vi "Get Limits.vi"(11 "Limits File Path":path=path "D:/PR002165_FCT_NGPMH/UTP/misc/Limits/Production_Limits.csv") -> (2 "DUT2":T1, 3 "DUT1":T1)   [LabVIEW 2023]
uses:
  DUT limits.ctl
  <vilib>/Utility/file.llb/Read Delimited Spreadsheet (DBL).vi
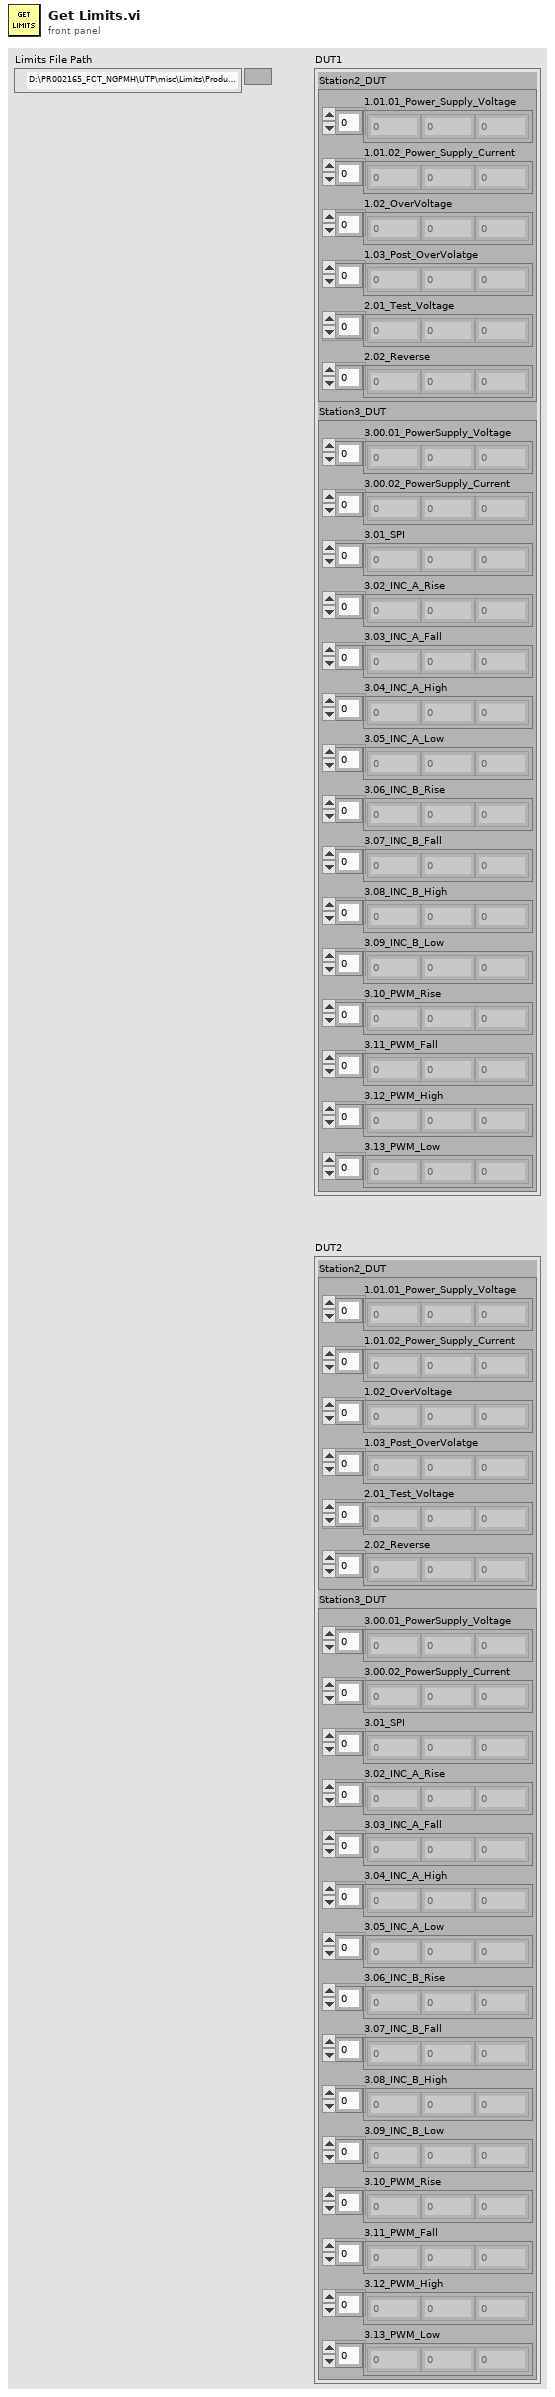
[diagram p1: front panel]
types:
  T1 = typedef "DUT limits.ctl" = cluster{"Station2_DUT":cluster{"1.01.01_Power_Supply_Voltage":dbl[], "1.01.02_Power_Supply_Current":dbl[], "1.02_OverVoltage":dbl[], "1.03_Post_OverVolatge":dbl[], "2.01_Test_Voltage":dbl[], "2.02_Reverse":dbl[]}, "Station3_DUT":cluster{"3.00.01_PowerSupply_Voltage":dbl[], "3.00.02_PowerSupply_Current":dbl[], "3.01_SPI":dbl[], "3.02_INC_A_Rise":dbl[], "3.03_INC_A_Fall":dbl[], "3.04_INC_A_High":dbl[], "3.05_INC_A_Low":dbl[], "3.06_INC_B_Rise":dbl[], "3.07_INC_B_Fall":dbl[], "3.08_INC_B_High":dbl[], "3.09_INC_B_Low":dbl[], "3.10_PWM_Rise":dbl[], "3.11_PWM_Fall":dbl[], "3.12_PWM_High":dbl[], "3.13_PWM_Low":dbl[]}}
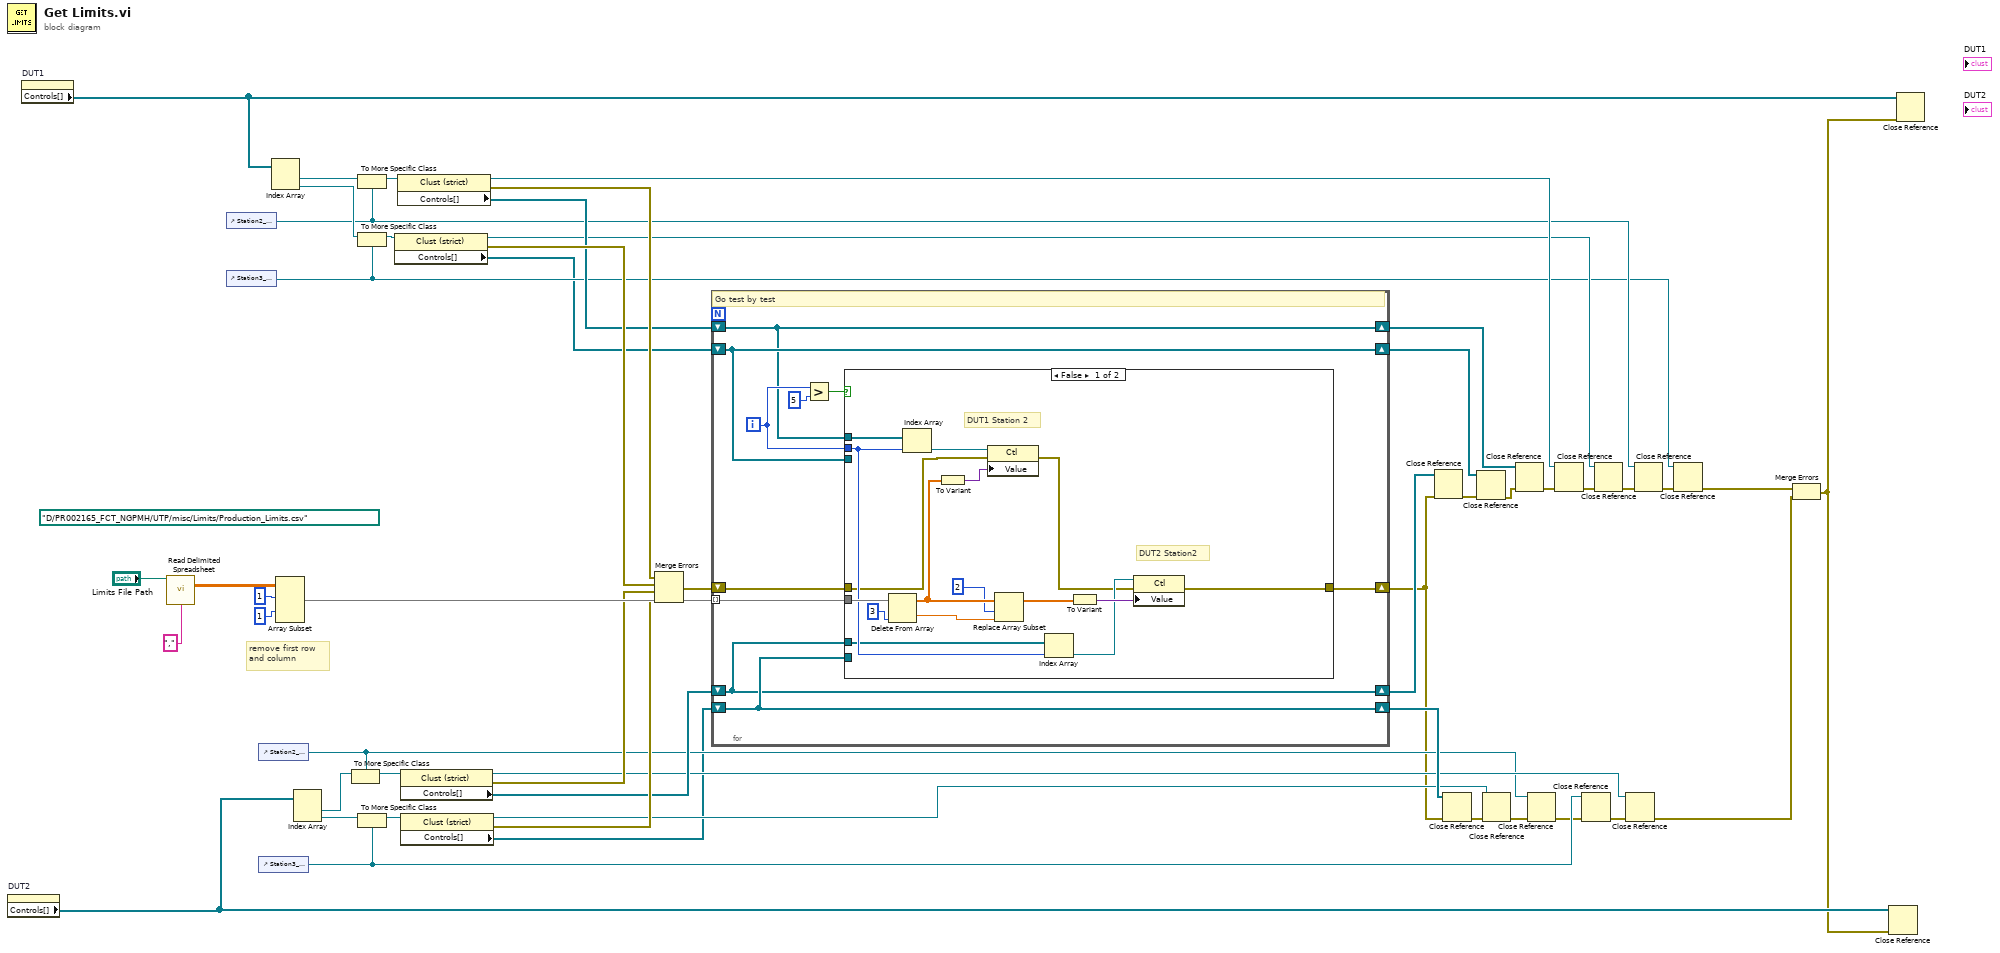
[diagram p0: block diagram]
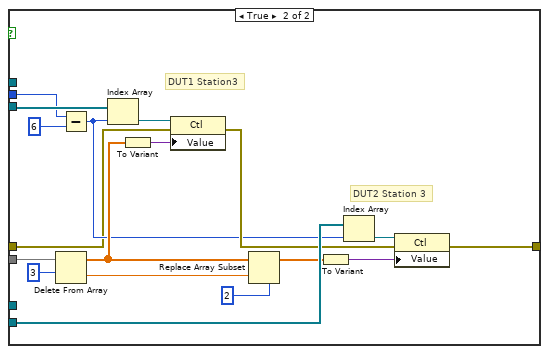
[diagram p2: hidden frame]
diagram:
  (unwired) path "D:/PR002165_FCT_NGPMH/UTP/misc/Limits/Production_Limits.csv" ("file path (dialog if empty)")
  # "remove first row\nand column"
  n1 = property on="DUT2" class="Clust (strict)"() -> ("Controls[]"=w27:refnum<vi>[])  [unwired: 2 in, 2 out]
  n2 = property on="DUT1" class="Clust (strict)"() -> ("Controls[]"=w11:refnum<vi>[])  [unwired: 2 in, 2 out]
  n3 = call-poly <vilib>:"Read Delimited Spreadsheet.vi"("file path (dialog if empty)"="Limits File Path", "delimiter (\\t)"="," ("delimiter (\\t)")) -> ("all rows"=w50:dbl[][])  [unwired: 8 in, 5 out]
  n4 = control-ref of="Station2_DUT"() -> (w19:refnum<vi>)
  n5 = control-ref of="Station3_DUT"() -> (w17:refnum<vi>)
  n6 = control-ref of="Station2_DUT"() -> (w15:refnum<vi>)
  n7 = control-ref of="Station3_DUT"() -> (w14:refnum<vi>)
  n8 = Index Array(array=w11) -> (element #1=w46:refnum<vi>, element #2=w44:refnum<vi>)  [unwired: 2 in]
  n9 = Array Subset(array=w50, index (row)=1 ("index"), index (col)=1 ("index")) -> (w48:dbl[][])  [unwired: 2 in]
  n10 = Index Array(array=w27) -> (element #1=w41:refnum<vi>, element #2=w40:refnum<vi>)  [unwired: 2 in]
  n11 = To More Specific Class(target class=w15, reference=w41) -> (specific class reference=w39:refnum<vi>)  [unwired: 1 in, 1 out]
  n12 = To More Specific Class(target class=w19, reference=w46) -> (specific class reference=w47:refnum<vi>)  [unwired: 1 in, 1 out]
  n13 = To More Specific Class(target class=w17, reference=w44) -> (specific class reference=w45:refnum<vi>)  [unwired: 1 in, 1 out]
  n14 = To More Specific Class(target class=w14, reference=w40) -> (specific class reference=w38:refnum<vi>)  [unwired: 1 in, 1 out]
  n15 = property class="Clust (strict)"(reference=w45) -> (reference out=w21:refnum<vi>, error out=w36:errorcluster, "Controls[]"=w5:refnum<vi>[])  [unwired: 1 in]
  n16 = property class="Clust (strict)"(reference=w47) -> (reference out=w23:refnum<vi>, error out=w37:errorcluster, "Controls[]"=w24:refnum<vi>[])  [unwired: 1 in]
  n17 = property class="Clust (strict)"(reference=w39) -> (reference out=w28:refnum<vi>, error out=w35:errorcluster, "Controls[]"=w33:refnum<vi>[])  [unwired: 1 in]
  n18 = property class="Clust (strict)"(reference=w38) -> (reference out=w29:refnum<vi>, error out=w34:errorcluster, "Controls[]"=w4:refnum<vi>[])  [unwired: 1 in]
  n19 = Merge Errors(w37, w36, w35, w34) -> (w9:errorcluster)
  n20 = for {
    tunnel: w48 -> [w61] mode=indexing
    shift-right: [w57] -> w43
    shift-left: w5 -> [w57]
    shift-right: [w56] -> w42
    shift-left: w24 -> [w56]
    shift-right: [w54] -> w32
    shift-left: w33 -> [w54]
    shift-right: [w55] -> w31
    shift-left: w4 -> [w55]
    shift-right: [w53] -> w6
    shift-left: w9 -> [w52]
    i -> [w58]
    # "Go test by test"
    n21 = Greater?(x=w58, y=5) -> (0:w59:bool)
    n22 = case shown="False" w59 {
      tunnel: w57 -> [_ w95]
      tunnel: w56 -> [w65 _]
      tunnel: w58 -> [w68 w90]
      tunnel: w61 -> [w71 w88]
      tunnel: w55 -> [_ w91]
      tunnel: w54 -> [w64 _]
      tunnel: [w63 w80] -> w53
      tunnel: w52 -> [w62 w78]
      frame False {
        # "DUT1 Station 2"
        # "DUT2 Station2"
        n23 = Delete From Array(array=w71, index=3 ("length")) -> (deleted portion=w73:dbl, array with subset deleted=w75:dbl[])  [unwired: 1 in]
        n24 = Index Array(array=w65, index=w68) -> (element=w77:refnum<vi>)
        n25 = To Variant(anything=w75) -> (Variant=w70:variant)
        n26 = property class="Ctl"(reference=w77, error in=w62, "Value"=w70) -> (error out=w66:errorcluster)  [unwired: 1 out]
        n27 = Replace Array Subset(array=w75, new element=w73, index=2) -> (w72:dbl[])
        n28 = Index Array(array=w64, index=w68) -> (element=w67:refnum<vi>)
        n29 = To Variant(anything=w72) -> (Variant=w69:variant)
        n30 = property class="Ctl"(reference=w67, error in=w66, "Value"=w69) -> (error out=w63:errorcluster)  [unwired: 1 out]
      }
      frame True {
        # "DUT1 Station3"
        # "DUT2 Station 3"
        n31 = Delete From Array(array=w88, index=3 ("length")) -> (deleted portion=w84:dbl, array with subset deleted=w86:dbl[])  [unwired: 1 in]
        n32 = Subtract(x=w90, y=6) -> (x-y=w79:i32)
        n33 = Index Array(array=w95, index=w79) -> (element=w93:refnum<vi>)
        n34 = To Variant(anything=w86) -> (Variant=w92:variant)
        n35 = property class="Ctl"(reference=w93, error in=w78, "Value"=w92) -> (error out=w81:errorcluster)  [unwired: 1 out]
        n36 = Replace Array Subset(array=w86, new element=w84, index=2) -> (w83:dbl[])
        n37 = To Variant(anything=w83) -> (Variant=w82:variant)
        n38 = Index Array(array=w91, index=w79) -> (element=w89:refnum<vi>)
        n39 = property class="Ctl"(reference=w89, error in=w81, "Value"=w82) -> (error out=w80:errorcluster)  [unwired: 1 out]
      }
    }
  }
  n40 = Close Reference(reference=w32, error in (no error)=w6) -> (error out=w7:errorcluster)
  n41 = Close Reference(reference=w31, error in (no error)=w6) -> (error out=w30:errorcluster)
  n42 = Close Reference(reference=w43, error in (no error)=w7) -> (error out=w8:errorcluster)
  n43 = Close Reference(reference=w29, error in (no error)=w30) -> (error out=w2:errorcluster)
  n44 = Close Reference(reference=w42, error in (no error)=w8) -> (error out=w22:errorcluster)
  n45 = Close Reference(reference=w15, error in (no error)=w2) -> (error out=w13:errorcluster)
  n46 = Close Reference(reference=w23, error in (no error)=w22) -> (error out=w20:errorcluster)
  n47 = Close Reference(reference=w14, error in (no error)=w13) -> (error out=w1:errorcluster)
  n48 = Close Reference(reference=w21, error in (no error)=w20) -> (error out=w18:errorcluster)
  n49 = Close Reference(reference=w28, error in (no error)=w1) -> (error out=w12:errorcluster)
  n50 = Close Reference(reference=w19, error in (no error)=w18) -> (error out=w16:errorcluster)
  n51 = Close Reference(reference=w17, error in (no error)=w16) -> (error out=w3:errorcluster)
  n52 = Merge Errors(w3, w12) -> (w10:errorcluster)
  n53 = Close Reference(reference=w27, error in (no error)=w10) -> ()  [unwired: 1 out]
  n54 = Close Reference(reference=w11, error in (no error)=w10) -> ()  [unwired: 1 out]
